vi "Move.vi"(8 "error in (no error)":errorcluster, 10 "Num Iterations":i32, 11 "BaseProducer in":refnum<class "BaseProducer.lvclass">) -> (0 "error out":errorcluster, 1 "Blow Out?":bool, 2 "Temperature Array (C)":dbl[](array[numeric]), 3 "BaseProducer out":refnum<class "BaseProducer.lvclass">)   [LabVIEW 2013, in "BaseProducer.lvclass"]
doc: "This method moves in a linearly-interpolated path to the next input target step."
uses:
  BaseProducer.lvclass
  BaseProducer.lvclass/BaseProducer.ctl
  <vilib>/DAQmx/write.llb/DAQmx Write (Analog 1D DBL NChan 1Samp).vi
  <vilib>/DAQmx/read.llb/DAQmx Read (Analog 1D DBL NChan 1Samp).vi
  <vilib>/DAQmx/read.llb/DAQmx Read (Analog 2D DBL NChan NSamp).vi
  <vilib>/DAQmx/miscellaneous.llb/DAQmx Fill In Error Info.vi
panel:
  in  "Skip Button":bool
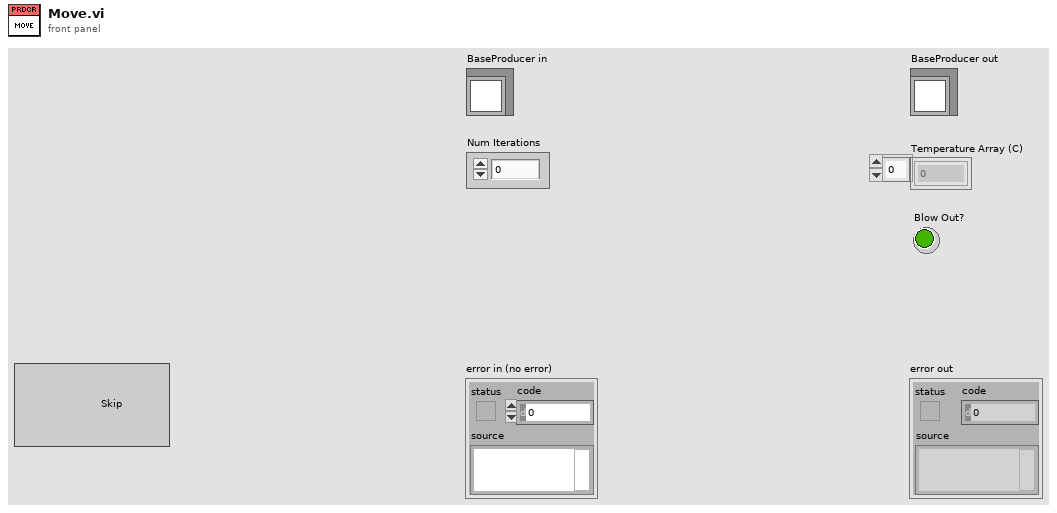
[diagram p1: front panel]
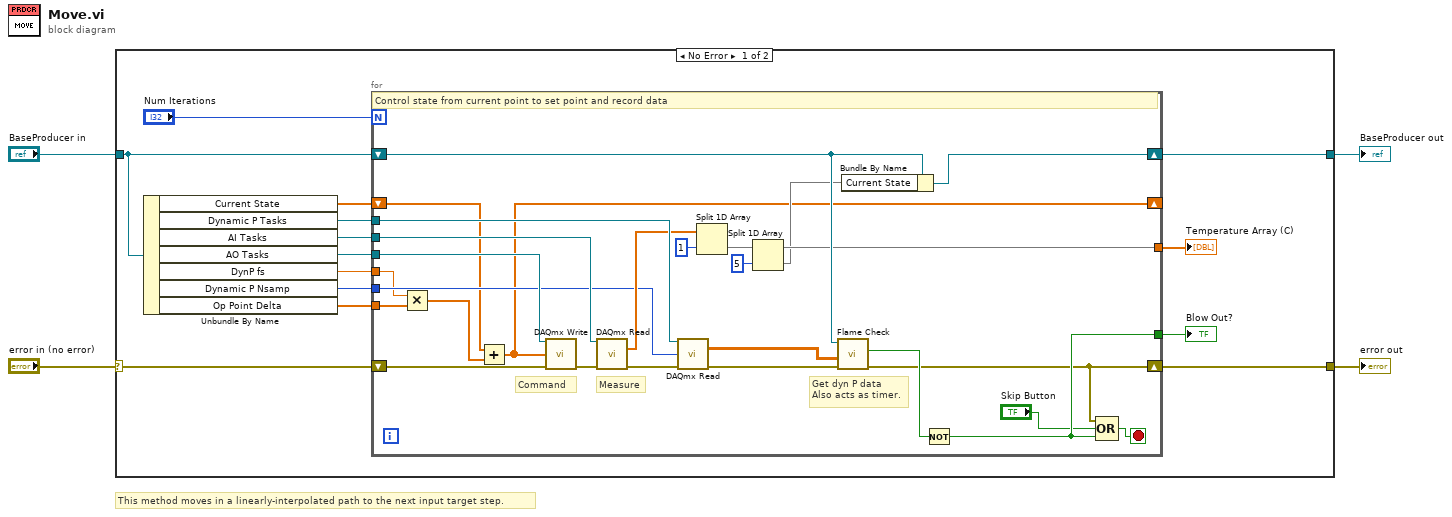
[diagram p0: block diagram]
diagram:
  # "This method moves in a linearly-interpolated path to the next input target step."
  n1 = case shown="No Error" "error in (no error)" {
    selector: "error in (no error)" -> [w18 w47]
    tunnel: [w17 w47] -> w2
    tunnel: [w9 w46] -> w1
    tunnel: "BaseProducer in" -> [w10 w46]
    frame No Error {
      n2 = Unbundle By Name(w10) -> ("Current State"=w5:dbl[], "Dynamic P Tasks"=w16:refnum<k21>, "AI Tasks"=w15:refnum<k21>, "AO Tasks"=w14:refnum<k21>, "DynP fs"=w13:dbl, "Dynamic P Nsamp"=w12:i32, "Op Point Delta"=w11:dbl[])
      n3 = for {
        N: "Num Iterations" -> [_]
        shift-right: [w19] -> w17
        shift-left: w18 -> [w45]
        tunnel: w16 -> [w40]
        tunnel: w14 -> [w44]
        tunnel: w15 -> [w43]
        tunnel: [w22] -> w6
        shift-right: [w24] -> w9
        shift-left: w10 -> [w32]
        tunnel: [w33] -> w7
        tunnel: w12 -> [w29]
        tunnel: w11 -> [w28]
        tunnel: w13 -> [w27]
        shift-right: [w20] -> _
        shift-left: w5 -> [w25]
        stop <- w31 stop-if-true
        # "Get dyn P data\nAlso acts as timer."
        # "Measure"
        # "Command"
        # "Control state from current point to set point and record data"
        n4 = Multiply(x=w27, y=w28) -> (x*y=w26:dbl[])
        n5 = Add(x=w25, y=w26) -> (x+y=w20:dbl[])
        n6 = call-poly <vilib>:"DAQmx Write.vi"("task/channels in"=w44, "data"=w20, "error in"=w45) -> ("error out"=w42:errorcluster)  [unwired: 10 in, 2 out]
        n7 = call-poly <vilib>:"DAQmx Read.vi"("task/channels in"=w43, "error in"=w42) -> ("data"=w39:dbl[], "error out"=w41:errorcluster)  [unwired: 11 in, 1 out]
        n8 = call-poly <vilib>:"DAQmx Read.vi"("task/channels in"=w40, "number of samples per channel"=w29, "error in"=w41) -> ("data"=w23:dbl[][], "error out"=w35:errorcluster)  [unwired: 10 in, 1 out]
        n9 = Split 1D Array(array=w39, index=1) -> (second subarray=w37:dbl[])  [unwired: 1 out]
        n10 = Split 1D Array(array=w37, index=5) -> (first subarray=w22:dbl[], second subarray=w21:dbl[])
        n11 = call "Flame Check.vi"("error in (no error)"=w35, "Dynamic P data"=w23, "BaseProducer in"=w32) -> ("error out"=w19:errorcluster, "Flame?"=w34:bool)  [unwired: 6 in, 1 out]
        n12 = Bundle By Name(cluster=w32, "Current State"=w21) -> (w24:refnum<class "BaseProducer.lvclass">)
        n13 = Not(x=w34) -> (.not. x?=w33:bool)
        n14 = Compound Arithmetic op=OR(w19, "Skip Button", w33) -> (w31:bool)
      }
      "Blow Out?" <- w7
      "Temperature Array (C)" <- w6
    }
    frame Error {
    }
  }
  "error out" <- w2
  "BaseProducer out" <- w1
